vi "Read Tab-Delimited File.vi"() -> ()   [LabVIEW 2023]
doc: "Reads a text file created by Write Tab-Delimited File.vi."
panel:
  out "Table of data":string[][](table)
  out "Raw Tab-Delimited Data":string
  out "Graph of data":dbl[][](graph)
  # "Overview: Demonstrates the use of the File I/O functions to read data from a tab-delimited text file.\nInstructions:\n1. Make sure you have already run Write Tab-Delimited File.vi.\n2. Run this VI. The contents of the file will be displayed in the Raw Tab-Delimited Data indicator below.\n3. Delete the text file (located at [LabVIEW Data]\\Example Tab-Delimited File.txt) when you are done."
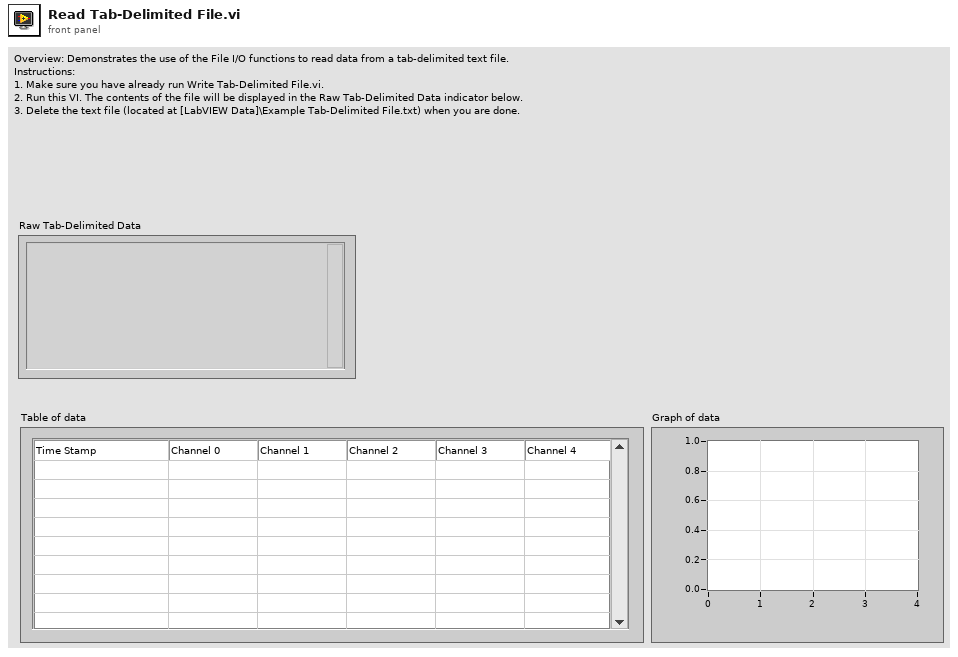
[diagram p1: front panel]
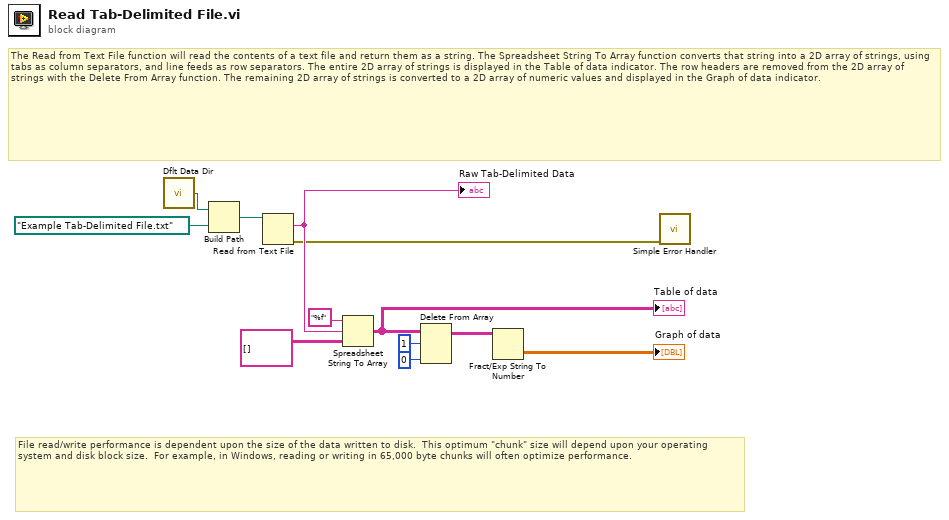
[diagram p0: block diagram]
diagram:
  # "File read/write performance is dependent upon the size of the data written to disk.  This optimum \"chunk\" size will depend upon your operating system and disk block size.  For example, in Windows, reading or writing in 65,000 byte chunks will often optimize performance."
  # "The Read from Text File function will read the contents of a text file and return them as a string. The Spreadsheet String To Array function converts that string into a 2D array of strings, using tabs as column separators, and line feeds as row separators. The entire 2D array of strings is displayed in the Table of data indicator. The row headers are removed from the 2D array of strings with the Delete From Array function. The remaining 2D array of strings is converted to a 2D array of numeric values and displayed in the Graph of data indicator."
  n1 = call <vilib>:"Dflt Data Dir.vi"() -> ("App:Default Data Directory"=w7:path)
  n2 = Build Path(base path=w7, name or relative path=path "Example Tab-Delimited File.txt" ("default name")) -> (appended path=w4:path)
  n3 = Read from Text File(file (use dialog)=w4) -> (text=w8:string, error out=w5:errorcluster)  [unwired: 2 in, 3 out]
  "Raw Tab-Delimited Data" <- w8
  n4 = Spreadsheet String To Array(format string="%f", spreadsheet string=w8, array type (2D Dbl)=string[][] [] ("Array")) -> (array=w1:string[][])  [unwired: 1 in]
  "Table of data" <- w1
  n5 = Delete From Array(array=w1, length=1, index (col)=0 ("disabled index (col)")) -> (array with subset deleted=w2:string[][])  [unwired: 1 in, 1 out]
  n6 = Fract/Exp String To Number(string=w2) -> (number=→"Graph of data":dbl[][])  [unwired: 4 out]
  n7 = call <vilib>:"Simple Error Handler.vi"("error in (no error)"=w5) -> ()  [unwired: 1 in, 8 out]
